vi "TestStaleInsertIntoPanel_Reject.vi"(8 "error in (no error)":errorcluster, 11 "TestCase in":refnum<class "TestProtectedSubpanel.lvclass">) -> (0 "error out":errorcluster, 3 "TestCase out":refnum<class "TestProtectedSubpanel.lvclass">)   [LabVIEW 2015, in "TestProtectedSubpanel.lvclass"]
uses:
  TestProtectedSubpanel.lvclass
  Framework/IViewable/ProtectedSubpanel/ProtectedSubpanel.lvclass
  <vilib>/addons/_JKI Toolkits/VI Tester/TestCase.llb/TestCase.lvclass
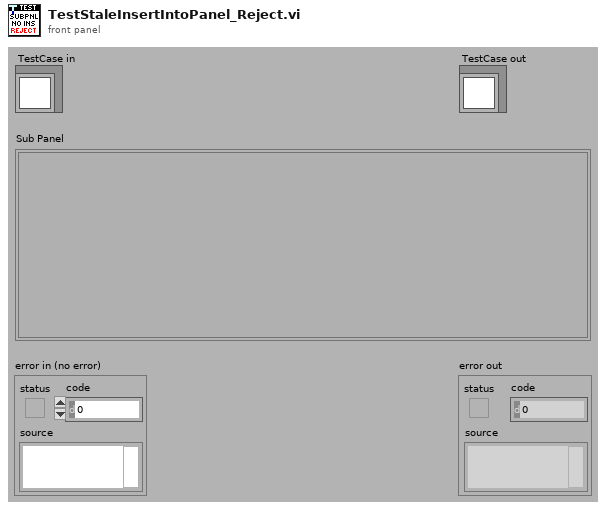
[diagram p1: front panel]
types:
  T1 = typedef "IViewable.lvlib/ProtectedSubpanel.lvclass/Protected Subpanel Reference.ctl" = refnum<data-value>
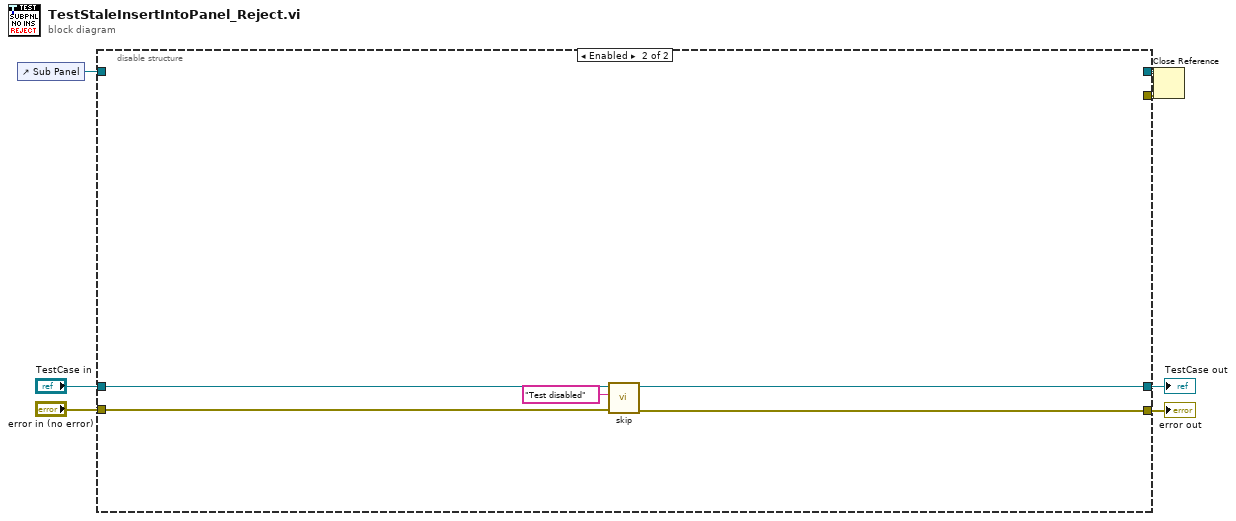
[diagram p0: block diagram]
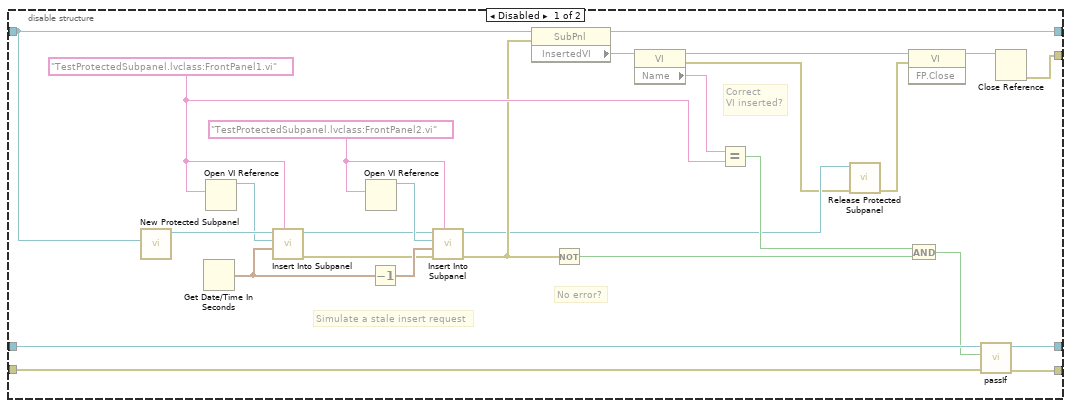
[diagram p2: hidden frame]
diagram:
  n1 = control-ref of="Sub Panel"() -> (w3:refnum<vi>)
  n2 = disable-structure shown="Enabled" {
    disable-tunnel: [w34 w36] -> w7
    disable-tunnel: "TestCase in" -> [w33 w39]
    disable-tunnel: [w32 w38] -> w5
    disable-tunnel: "error in (no error)" -> [w31 w37]
    disable-tunnel: w3 -> [w17 _]
    disable-tunnel: [w14 _] -> w2
    disable-tunnel: [w10 _] -> w1
    frame Disabled {
      w23 = "TestProtectedSubpanel.lvclass:FrontPanel2.vi"
      w21 = "TestProtectedSubpanel.lvclass:FrontPanel1.vi"
      # "Simulate a stale insert request"
      # "No error?"
      # "Correct\nVI inserted?"
      n3 = call "New Protected Subpanel.vi"("SubPnl Refnum"=w17) -> ("Protected Subpanel"=w30:T1)  [unwired: 9 in, 1 out]
      n4 = Get Date/Time In Seconds() -> (seconds since 1Jan1904=w19:timestamp)
      n5 = Open VI Reference(vi path=w21) -> (vi reference=w29:refnum<vi>)  [unwired: 5 in, 1 out]
      n6 = call "Insert Into Subpanel.vi"(7:w21, "Insertion Request Time"=w19, "Viewable"=w29, "Protected Subpanel"=w30) -> ("error out"=w16:errorcluster, "Protected Subpanel"=w20:T1)  [unwired: 4 in, 2 out]
      n7 = Open VI Reference(vi path=w23) -> (vi reference=w22:refnum<vi>)  [unwired: 5 in, 1 out]
      n8 = Decrement(x=w19) -> (x-1=w18:timestamp)
      n9 = call "Insert Into Subpanel.vi"(7:w23, "error in (no error)"=w16, "Insertion Request Time"=w18, "Viewable"=w22, "Protected Subpanel"=w20) -> ("error out"=w15:errorcluster, "Protected Subpanel"=w12:T1)  [unwired: 3 in, 2 out]
      n10 = property class="SubPnl"(reference=w17, error in=w15) -> (reference out=w14:refnum<vi>, "InsertedVI"=w27:refnum<vi>)  [unwired: 1 out]
      n11 = Not(x=w15) -> (.not. x?=w28:bool)
      n12 = property class="VI"(reference=w27) -> (reference out=w13:refnum<vi>, error out=w11:errorcluster, "Name"=w25:string)  [unwired: 1 in]
      n13 = Equal?(x=w25, y=w21) -> (x = y?=w24:bool)
      n14 = call "Release Protected Subpanel.vi"("error in (no error)"=w11, "Protected Subpanel"=w12) -> ("error out"=w8:errorcluster)  [unwired: 9 in]
      n15 = invoke class="VI" method="FP.Close"(reference=w13, error in=w8) -> (reference out=w9:refnum<vi>)  [unwired: 1 in, 2 out]
      n16 = And(x=w24, y=w28) -> (x .and. y?=w26:bool)
      n17 = call-dynamic "passIf.vi"("error in (no error)"=w31, "pass"=w26, "TestCase in"=w33) -> ("error out"=w34:errorcluster, "TestCase out"=w32:refnum<class "TestProtectedSubpanel.lvclass">)  [unwired: 7 in]
      n18 = Close Reference(reference=w9) -> (error out=w10:errorcluster)  [unwired: 1 in]
    }
    frame Enabled {
      n19 = call <vilib>:"skip.vi"("error in (no error)"=w37, "skipMessage"="Test disabled", "TestCase in"=w39) -> ("error out"=w36:errorcluster, "TestCase out"=w38:refnum<class "TestProtectedSubpanel.lvclass">)  [unwired: 7 in]
    }
  }
  "error out" <- w7
  "TestCase out" <- w5
  n20 = Close Reference(reference=w2, error in (no error)=w1) -> ()  [unwired: 1 out]
